vi "RDB Parse.vi"(8 "error in (no error)":errorcluster, 10 "RDB Message":string, 11 "Settings":T1={"UDP Receiver"=refnum, "UDP Sender"=refnum, "Valid Packet"=FALSE, "TCP"=refnum, "Network Settings"={"IP adress"="127.0.0.1", "RDB"={"Protocol"=enum."UDP", "Tx Port"=48270, "Rx Port"=10, "Buffer Size"=204800, "Timeout"=10}, "SCP"={"Protocol"=enum."TCP", "Tx Port"=48191, "Rx Port"=48191, "Buffer Size"=204800, "Timeout"=10}}, "vclient"=path ""}) -> (0 "error out":errorcluster, 2 "Status":dbl[](array[numeric]), 3 "Settings":T1={"UDP Receiver"=refnum, "UDP Sender"=refnum, "Valid Packet"=FALSE, "TCP"=refnum, "Network Settings"={"IP adress"="127.0.0.1", "RDB"={"Protocol"=enum."UDP", "Tx Port"=48270, "Rx Port"=10, "Buffer Size"=204800, "Timeout"=10}, "SCP"={"Protocol"=enum."TCP", "Tx Port"=48191, "Rx Port"=48191, "Buffer Size"=204800, "Timeout"=10}}, "vclient"=path ""})   [LabVIEW 2020, in "RDB.lvlib"]
uses:
  RDB.lvlib
  Engine/Type/Settings.ctl
  Shared/Network Settings.ctl
  Shared/Protocol.ctl
  Engine/Vires VTD Engine.lvlib
  Shared/Vires VTD Shared.lvlib
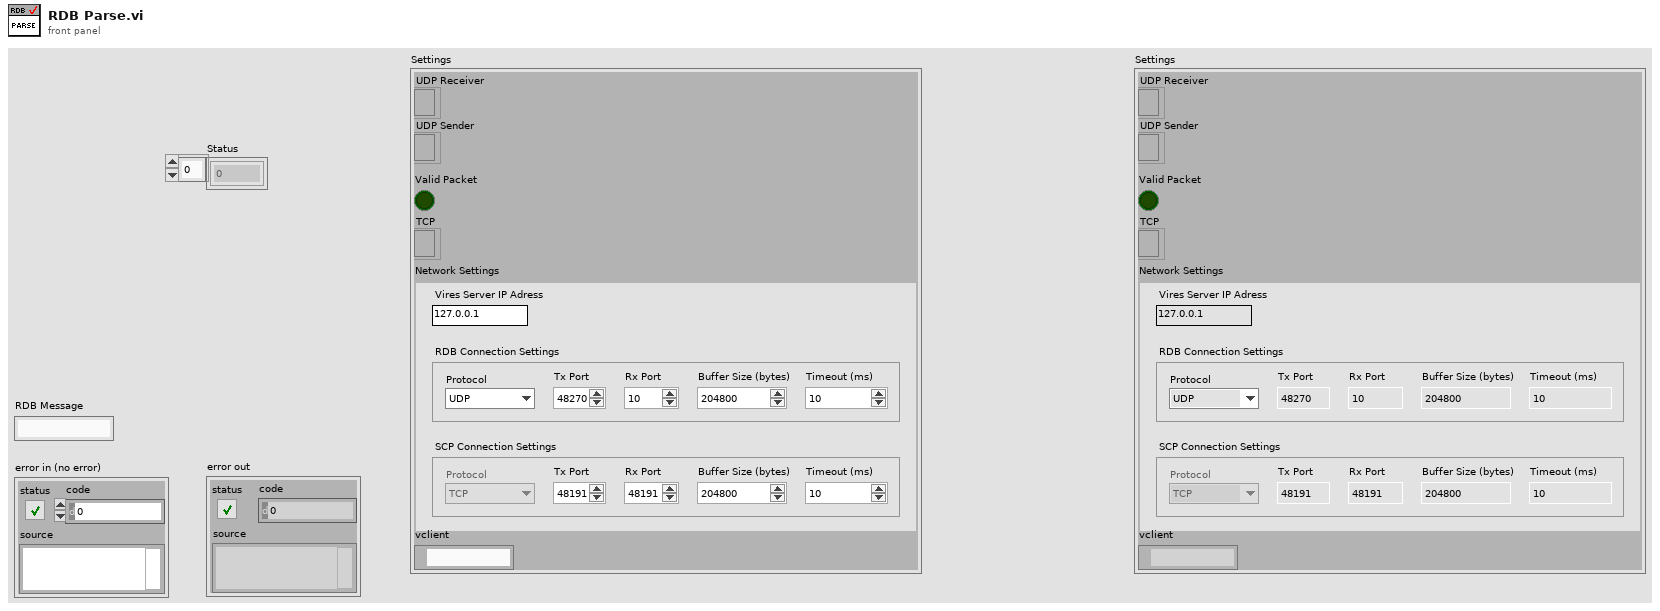
[diagram p1: front panel]
types:
  T1 = typedef "Vires VTD Engine.lvlib/Settings.ctl" = cluster{"UDP Receiver":refnum<k16>, "UDP Sender":refnum<k16>, "Valid Packet":bool, "TCP":refnum<k5>, "Network Settings":T2, "vclient":path}
  T2 = typedef "Vires VTD Shared.lvlib/Network Settings.ctl" = cluster{"IP adress":string, "RDB":cluster{"Protocol":T3, "Tx Port":u16, "Rx Port":u16, "Buffer Size":i32, "Timeout":u16}, "SCP":cluster{"Protocol":T3, "Tx Port":u16, "Rx Port":u16, "Buffer Size":i32, "Timeout":u16}}
  T3 = typedef "Vires VTD Shared.lvlib/Protocol.ctl" = enum16{"UDP", "TCP"}
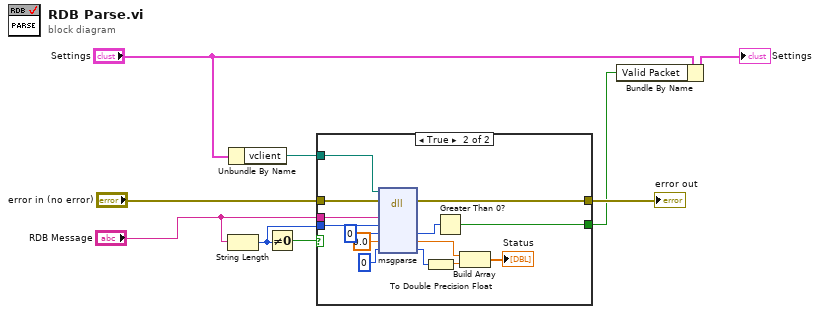
[diagram p0: block diagram]
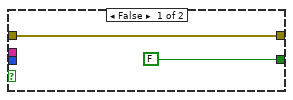
[diagram p2: hidden frame]
diagram:
  n1 = String Length(string="RDB Message") -> (length=w3:i32)
  n2 = Unbundle By Name("Settings") -> ("vclient"=w2:path)
  n3 = Not Equal To 0?(x=w3) -> (x != 0?=w6:bool)
  n4 = case shown="True" w6 {
    tunnel: "error in (no error)" -> [w11 w25]
    tunnel: [w11 w24] -> w8
    tunnel: "RDB Message" -> [_ w23]
    tunnel: [FALSE w20] -> w4
    tunnel: w3 -> [_ w19]
    tunnel: w2 -> [_ w18]
    frame False {
    }
    frame True {
      n5 = dll-call lib="E:/Documents/Systems Engineering/Custom VeriStand Development/Vires VTD Custom Device/Vires VTD Custom Device/Vires VTD/Source/RDB/vclient.*" fn="msgparse"(path in=w18, error in=w25, "RDBmessage"=w23, "size"=w19, "valid"=u8 0, "simTime"=0.0, "simFrame"=0) -> (error out=w24:errorcluster, "valid"=w21:u8, "simTime"=w14:dbl, "simFrame"=w15:i32)  [unwired: 4 in, 1 out]
      n6 = To Double Precision Float(number=w15) -> (double precision float=w13:dbl)
      n7 = Greater Than 0?(x=w21) -> (x > 0?=w20:bool)
      n8 = Build Array(w14, w13) -> (→"Status":dbl[])
    }
  }
  "error out" <- w8
  n9 = Bundle By Name(cluster="Settings", "Valid Packet"=w4) -> (→"Settings":T1)
